vi "Create NotifyIcon.vi"(4 "error in (no error)":errorcluster) -> (0 "error out":errorcluster, 3 "NotifyIcon":refnum<k24>)   [LabVIEW 2014, in "NotifyIcon.lvlib"]
uses:
  NotifyIcon.lvlib
  System.Windows.Forms
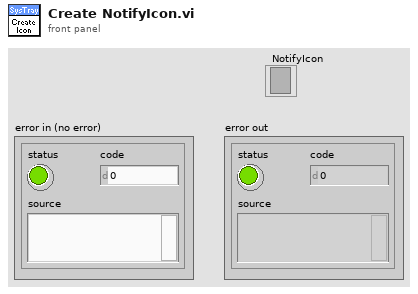
[diagram p1: front panel]
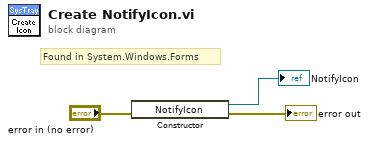
[diagram p0: block diagram]
diagram:
  # "Found in System.Windows.Forms"
  n1 = constructor class="NotifyIcon"(error in="error in (no error)") -> (reference out=→"NotifyIcon":refnum<k24>, error out=→"error out":errorcluster)  [unwired: 2 in, 1 out]
